vi "FTW-Test-JSON-Parallelization.vi"() -> (0 "Test Result":errorcluster)   [LabVIEW 2015]
uses:
  src/time/FTW-Time-RelativeTimer.vi
  source/JSON/FTW-JSON-JoinMode.ctl
  source/Error/FTW-ERR-ExceptionType.ctl
  codegen/xnode/FTW-JSON-Fetch.xnode
  codegen/xnode/FTW-Dataflow-Synchronizer.xnode
  source/JSON/FTW-JSON-Core-LibraryFilepath.vi
  source/Error/FTW-ERR-ThrowError.vi
  source/CodeGen/JSON Deserialize/FTW-JSON-Core-GetFlattenedValue.vi
  source/Reflection/FTW-Reflection-Type.vi
  source/JSON/core/FTW-JSON-Core-EncodingFlags.vi
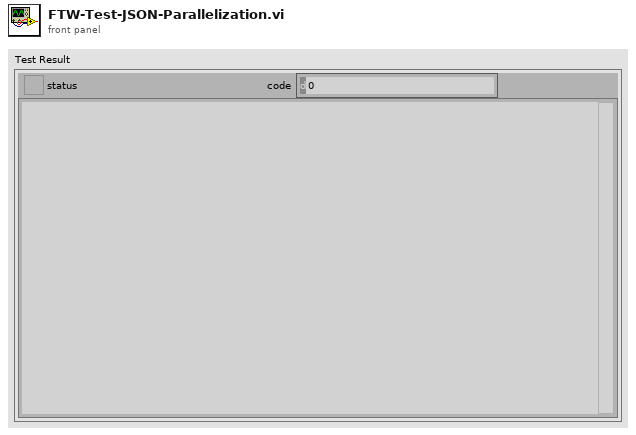
[diagram p1: front panel]
types:
  T1 = cluster{"LoggerDirectory":path, "Value":dbl, "LoggerAddress":string, "BooleanTrue":bool}
  T2 = typedef "FTW-ERR-ExceptionType.ctl" = enum16{"No Error", "Error", "Warning"}
  T3 = typedef "FTW-JSON-JoinMode.ctl" = enum32{"Upsert", "Update Only", "Insert Only"}
  T4 = typedef "FTW-Type-JSON.ctl" = refnum<data-value>
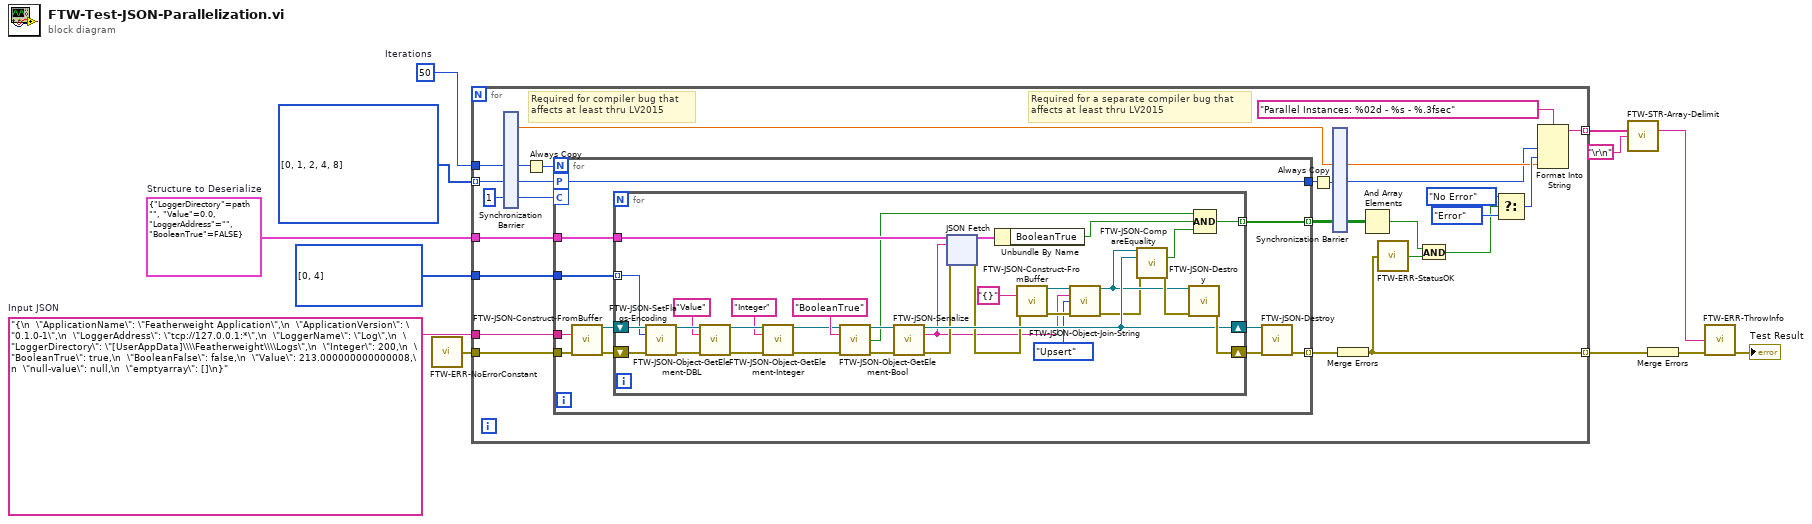
[diagram p0: block diagram]
diagram:
  w8 = T1 {"LoggerDirectory"=path "", "Value"=0.0, "LoggerAddress"="", "BooleanTrue"=FALSE}  # Structure to Deserialize
  w12 = "{\n  \"ApplicationName\": \"Featherweight Application\",\n  \"ApplicationVersion\": \"0.1.0-1\",\n  \"LoggerAddress\": \"tcp://127.0.0.1:*\",\n  \"LoggerName\": \"Log\",\n  \"LoggerDirectory\": \"[UserAppData]\\\\Featherweight\\\\Logs\",\n  \"Integer\": 200,\n  \"BooleanTrue\": true,\n  \"BooleanFalse\": false,\n  \"Value\": 213.000000000000008,\n  \"null-value\": null,\n  \"emptyarray\": []\n}"  # Input JSON
  w6 = 50  # Iterations
  n1 = call "FTW-ERR-NoErrorConstant.vi"() -> ("no error"=w11:errorcluster)
  n2 = for {
    tunnel: w6 -> [w28]
    tunnel: w12 -> [w40]
    tunnel: w11 -> [w39]
    tunnel: i32[] [0, 4] -> [w22]
    tunnel: i32[] [0, 1, 2, 4, 8] -> [w26] mode=indexing
    tunnel: w8 -> [w35]
    tunnel: [w33] -> w3 mode=indexing
    tunnel: [w32] -> w7 mode=indexing
    # "Required for a separate compiler bug that\naffects at least thru LV2015"
    # "Required for compiler bug that\naffects at least thru LV2015"
    n3 = xnode "Synchronization Barrier"("Synchronized Signal 1"=w28, "Synchronized Signal 3"=w26, 1) -> ("High-Resolution Timer"=w24:dbl, "Iterations out"=w27:i32, "Parallel Instances out"=w25:i32, "out"=w18:i32)  [unwired: 3 in, 1 out]
    n4 = Always Copy(1:w27) -> (0:w14:i32)
    n5 = for {
      N: w14 -> [_]
      tunnel: w40 -> [w60]
      tunnel: [w54] -> w17 mode=indexing
      tunnel: w22 -> [w55]
      workers-P: w25 -> [w53]
      tunnel: w39 -> [w62]
      tunnel: [w61] -> w38 mode=indexing
      tunnel: [w53] -> w21
      tunnel: w35 -> [w52]
      chunk-C: w18 -> [_]
      n6 = call "FTW-JSON-Construct-FromBuffer.vi"("JSON String (UTF-8)"=w60, "error in"=w62) -> ("JSON"=w56:refnum<class "FTW-Container.lvclass">, "error out"=w57:errorcluster)  [unwired: 12 in]
      n7 = for {
        tunnel: w55 -> [w90] mode=indexing
        shift-right: [w89] -> w58
        shift-left: w56 -> [w91]
        shift-right: [w94] -> w59
        shift-left: w57 -> [w92]
        tunnel: [w83] -> w54 mode=indexing
        tunnel: w52 -> [w86]
        n8 = call "FTW-JSON-SetFlags-Encoding.vi"("JSON"=w91, "Indent Spaces"=w90, "error in"=w92) -> ("JSON out"=w85:refnum<class "FTW-Container.lvclass">, "error out"=w84:errorcluster)  [unwired: 11 in]
        n9 = call "FTW-JSON-Object-GetElement-DBL.vi"("JSON"=w85, "Key"="Value", "error in"=w84) -> ("JSON out"=w70:refnum<class "FTW-Container.lvclass">, "error out"=w68:errorcluster)  [unwired: 9 in, 2 out]
        n10 = call "FTW-JSON-Object-GetElement-Integer.vi"("JSON"=w70, "Key"="Integer", "error in"=w68) -> ("JSON out"=w69:refnum<class "FTW-Container.lvclass">, "error out"=w67:errorcluster)  [unwired: 9 in, 2 out]
        n11 = call "FTW-JSON-Object-GetElement-Bool.vi"("JSON"=w69, "Key"="BooleanTrue", "error in"=w67) -> ("JSON out"=w82:refnum<class "FTW-Container.lvclass">, "Value"=w71:bool, "error out"=w81:errorcluster)  [unwired: 9 in, 1 out]
        n12 = call "FTW-JSON-Serialize.vi"("JSON"=w82, "error in"=w81) -> ("JSON out"=w89:refnum<class "FTW-Container.lvclass">, "JSON String (UTF-8)"=w73:string, "error out"=w88:errorcluster)  [unwired: 11 in]
        n13 = xnode "JSON Fetch"("Type and Defaults"=w86, "JSON String"=w73, "error in"=w88) -> ("Values"=w64:T1, "error out"=w87:errorcluster)  [unwired: 1 in]
        n14 = Unbundle By Name(w64) -> ("BooleanTrue"=w63:bool)
        n15 = call "FTW-JSON-Construct-FromBuffer.vi"("JSON String (UTF-8)"="{}", "error in"=w87) -> ("JSON"=w77:refnum<class "FTW-Container.lvclass">, "error out"=w75:errorcluster)  [unwired: 12 in]
        n16 = call "FTW-JSON-Object-Join-String.vi"("JSON"=w77, "JSON String to Join"=w73, "Update Mode"=FTW-JSON-JoinMode."Upsert", "error in"=w75) -> ("JSON out"=w76:T4, "error out"=w74:errorcluster)  [unwired: 10 in]
        n17 = call "FTW-JSON-CompareEquality.vi"("JSON"=w76, "JSON to Compare"=w89, "error in"=w74) -> ("Equal?"=w65:bool, "error out"=w93:errorcluster)  [unwired: 11 in]
        n18 = call "FTW-JSON-Destroy.vi"("JSON"=w76, "error in"=w93) -> ("error out"=w94:errorcluster)  [unwired: 13 in]
        n19 = Compound Arithmetic op=AND(w71, w63, w65) -> (w83:bool)
      }
      n20 = call "FTW-JSON-Destroy.vi"("JSON"=w58, "error in"=w59) -> ("error out"=w61:errorcluster)  [unwired: 13 in]
    }
    n21 = Always Copy(1:w21) -> (0:w13:i32)
    n22 = xnode "Synchronization Barrier"("Upstream Timer Value"=w24, "Synchronized Signal 6"=w13, w17) -> ("Elapsed Time"=w23:dbl, "out"=w20:i32, "out"=w16:bool[][])  [unwired: 4 in, 1 out]
    n23 = Merge Errors(w38) -> (w32:errorcluster)
    n24 = And Array Elements(Boolean array=w16) -> (logical AND=w36:bool)
    n25 = call "FTW-ERR-StatusOK.vi"("error to check"=w32) -> ("Status OK?"=w37:bool)
    n26 = And(x=w36, y=w37) -> (x .and. y?=w29:bool)
    n27 = Select(t=FTW-ERR-ExceptionType."No Error" ("Exception"), s=w29, f=FTW-ERR-ExceptionType."Error" ("Exception")) -> (s? t:f=w34:T2)
    n28 = Format Into String(format string="Parallel Instances: %02d - %s - %.3fsec", w20, w34, w23) -> (resulting string=w33:string)  [unwired: 2 in, 1 out]
  }
  n29 = call "FTW-STR-Array-Delimit.vi"("Array of Strings"=w3, "Delimiter"="\r\n") -> ("Delimited String"=w2:string)  [unwired: 13 in]
  n30 = Merge Errors(w7) -> (w5:errorcluster)
  n31 = call "FTW-ERR-ThrowInfo.vi"("Informational Message"=w2, "error in"=w5) -> ("error out"=→"Test Result":errorcluster)  [unwired: 13 in]
